vi "Set HW Interface Inputs.vi"(8 "error in (no error)":errorcluster, 9 "Digital Inputs":T1, 10 "Analog Inputs":T2, 11 "Grips Robot in":refnum<class "Grips Robot.lvclass">) -> (0 "error out":errorcluster, 3 "Grips Robot out":refnum<class "Grips Robot.lvclass">)   [LabVIEW 2013, in "Grips Robot.lvclass"]
uses:
  Grips Robot.lvclass
  Hardware Interface/DblArrayWithName.ctl
  Hardware Interface/BoolArrayWithName.ctl
  Grips Robot.lvclass/Grips Robot.ctl
  Hardware Interface/Hardware Interface.lvclass/Hardware Interface.ctl
  Hardware Interface/Hardware Interface.lvclass
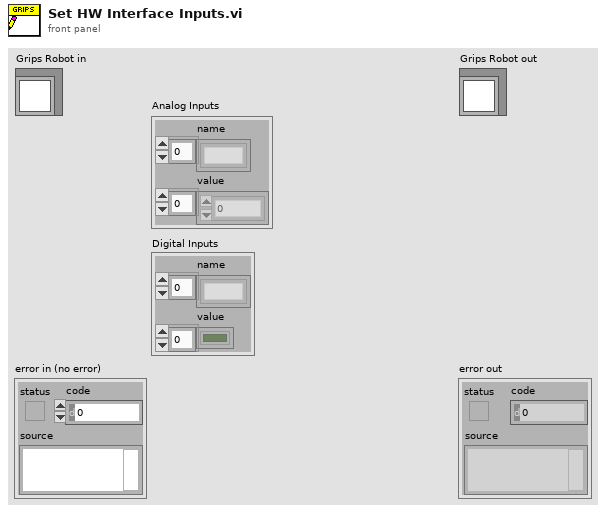
[diagram p1: front panel]
types:
  T1 = typedef "Hardware Interface.lvclass/BoolArrayWithName.ctl" = cluster{"name":string[], "value":bool[]}
  T2 = typedef "Hardware Interface.lvclass/DblArrayWithName.ctl" = cluster{"name":string[], "value":dbl[]}
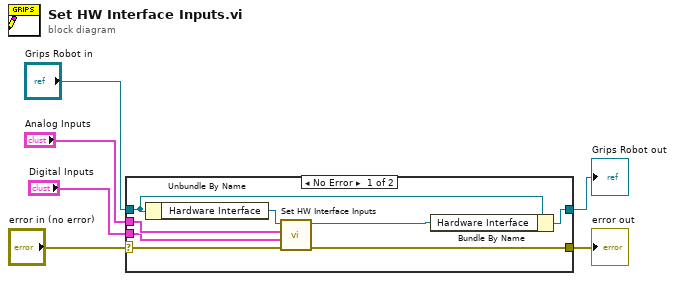
[diagram p0: block diagram]
diagram:
  n1 = case shown="No Error" "error in (no error)" {
    selector: "error in (no error)" -> [w10 w15]
    tunnel: [w9 w15] -> w5
    tunnel: [w14 w16] -> w3
    tunnel: "Grips Robot in" -> [w13 w16]
    tunnel: "Analog Inputs" -> [w8 _]
    tunnel: "Digital Inputs" -> [w7 _]
    frame No Error {
      n2 = Unbundle By Name(w13) -> ("Hardware Interface"=w12:refnum<class "Hardware Interface.lvclass">)
      n3 = call "Set HW Interface Inputs.vi"("error in (no error)"=w10, "Digital Inputs"=w7, "Analog Inputs"=w8, "Hardware Interface in"=w12) -> ("error out"=w9:errorcluster, "Hardware Interface out"=w11:refnum<class "Hardware Interface.lvclass">)  [unwired: 6 in]
      n4 = Bundle By Name(cluster=w13, "Hardware Interface"=w11) -> (w14:refnum<class "Grips Robot.lvclass">)
    }
    frame Error {
    }
  }
  "error out" <- w5
  "Grips Robot out" <- w3
